vi "Type Code to PV Name.vi"(8 "error in (no error)":errorcluster, 11 "type code":T1) -> (0 "error out":errorcluster, 3 "PV name":string)   [LabVIEW 2020]
uses:
  <vilib>/regexp/Match Regular Expression.xnode
  <userlib>/_OpenG.lib/lvdata/lvdata.llb/openg_variant.lvlib
  source/Value/Type Code.ctl
  source/Value/Value.lvlib
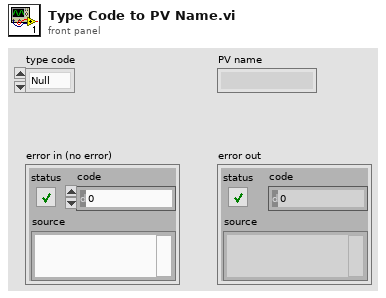
[diagram p1: front panel]
types:
  T1 = typedef "Value.lvlib/Type Code.ctl" = enum8{"Null", "Bool", "BoolA", "Int8", "Int8A", "Int16", "Int16A", "Int32", "Int32A", "Int64", "Int64A", "UInt8", "UInt8A", "UInt16", "UInt16A", "UInt32", "UInt32A", "UInt64", "UInt64A", "Float32", "Float32A", "Float64", "Float64A", "String", "StringA", "Struct", "StructA", "Union", "UnionA", "Any", "AnyA"}
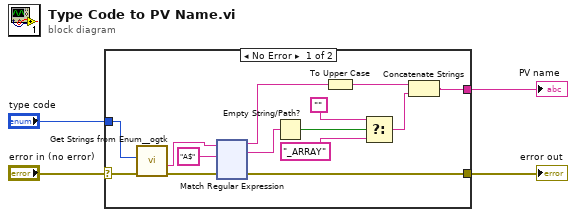
[diagram p0: block diagram]
diagram:
  n1 = case shown="No Error" "error in (no error)" {
    selector: "error in (no error)" -> [w17 w136]
    tunnel: [w18 w136] -> w4
    tunnel: "type code" -> [w6 _]
    tunnel: [w5 _] -> w2
    frame No Error {
      n2 = call <userlib>:"Get Strings from Enum__ogtk.vi"("error in (no error)"=w17, "Enum"=w6) -> ("error out"=w8:errorcluster, "String Value"=w7:string)  [unwired: 6 in, 2 out]
      n3 = xnode "Match Regular Expression"("input string"=w7, "regular expression"="A$", "error in"=w8) -> ("before match"=w9:string, "whole match"=w15:string, "error out"=w18:errorcluster)  [unwired: 3 in, 2 out]
      n4 = Empty String/Path?(string/path=w15) -> (empty?=w14:bool)
      n5 = To Upper Case(1:w9) -> (0:w10:string)
      n6 = Select(t="", s=w14, f="_ARRAY" ("regular expression")) -> (s? t:f=w12:string)
      n7 = Concatenate Strings(w10, w12) -> (w5:string)
    }
    frame Error {
    }
  }
  "error out" <- w4
  "PV name" <- w2
